vi "Write TDMS_Path.vi"(8 "error in":errorcluster, 10 "TDMS_Path":path, 11 "Report Viewer in":refnum<class "Report Viewer.lvclass">) -> (0 "error out":errorcluster, 3 "Report Viewer out":refnum<class "Report Viewer.lvclass">)   [LabVIEW 2023, in "Report Viewer.lvlib" / "Report Viewer.lvclass"]
uses:
  Library/Report Viewer.lvclass
  Library/Report Viewer.lvclass/Report Viewer.ctl
  Write tdms file ref.vi
  Private/Tree/Insert File Content.vi
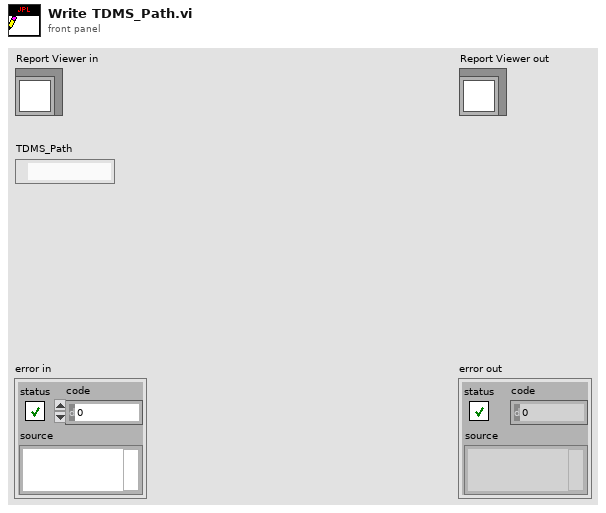
[diagram p1: front panel]
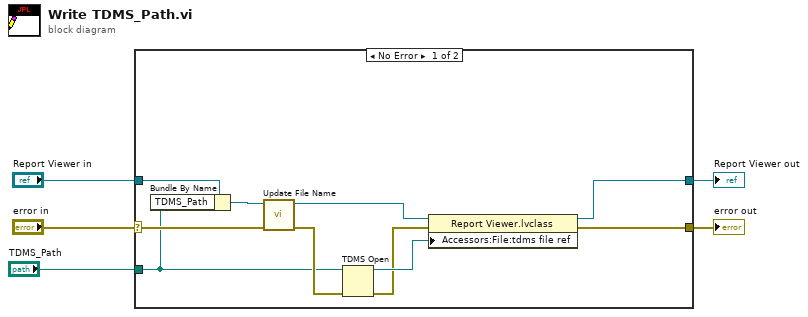
[diagram p0: block diagram]
diagram:
  n1 = case shown="No Error" "error in" {
    selector: "error in" -> [w11 w16]
    tunnel: [w9 w16] -> w4
    tunnel: [w7 w17] -> w2
    tunnel: "Report Viewer in" -> [w12 w17]
    tunnel: "TDMS_Path" -> [w6 _]
    frame No Error {
      n2 = Bundle By Name(cluster=w12, "TDMS_Path"=w6) -> (w13:refnum<class "Report Viewer.lvclass">)
      n3 = call "Update File Name.vi"("error in"=w11, "Report Viewer in"=w13) -> ("error out"=w10:errorcluster, "Report Viewer out"=w8:refnum<class "Report Viewer.lvclass">)  [unwired: 8 in]
      n4 = TDMS Open(8:w10, 11:w6) -> (0:w14:errorcluster, 3:w15:refnum<k34>)  [unwired: 5 in]
      n5 = property class="Report Viewer.lvclass"(reference=w8, error in=w14, "Accessors:File:tdms file ref"=w15) -> (reference out=w7:refnum<class "Report Viewer.lvclass">, error out=w9:errorcluster)
    }
    frame Error {
    }
  }
  "error out" <- w4
  "Report Viewer out" <- w2
